vi "AUTO - TRANSLATE.vi"(8 "error in (no error)":errorcluster, 11 "auto pgm step":T2={"auto drive command"={"TRANSLATE"={"drive\ndistance (ft)"=0.0, "steer\nbearing (deg)"=0.0, "max strafe\nvelocity (ft/s)"=0.0, "max strafe\naccel (ft/s^2)"=58.7}, "ROTATE"={"rotate to\nbearing (deg)"=0.0, "max rotate\nvelocity (deg/s)"=0.0, "max rotate\naccel (ft/s^2)"=25.0}}, "sub-systems"={"start INTAKE"=FALSE, "extend FLAP"=FALSE, "SHOOT"=FALSE, "retract FLAP"=FALSE, "TARGET SPEAKER"=FALSE, "TARGET AMP"=FALSE, "TARGET OFF"=FALSE, "DANCE"=FALSE}} {"auto drive command"."ROTATE"."max rotate\naccel (ft/s^2)" min=0.0 max=200.0 step=0.1 format="%_3f"; "auto drive command"."ROTATE"."max rotate\nvelocity (deg/s)" min=0.0 step=0.001; "auto drive command"."TRANSLATE"."max strafe\naccel (ft/s^2)" min=0.0 max=200.0 step=0.1 format="%_3f"; "auto drive command"."TRANSLATE"."max strafe\nvelocity (ft/s)" min=0.0 max=20.0 step=0.001 format="%_5f"}) -> (0 "error out":errorcluster)   [LabVIEW 2023]
uses:
  ctrl defs/ctrl AUTONOMOUS step control.ctl
  ctrl defs/ctrl AUTONOMOUS drive step control.ctl
  ctrl defs/ctrl AUTONOMOUS systems step control.ctl
  <vilib>/Rock Robotics/WPI/ThirdParty/REV Robotics/REVLib/Typedef/Spark MAX Control Type.ctl
  Global INIT.vi
  Global odometry.vi
  <vilib>/addons/control/pid/pid.llb/PID (DBL).vi
  <vilib>/Rock Robotics/WPI/ThirdParty/Phoenix-LabVIEW/CANCoder/Get/CTRE_Phoenix_CANcoder_GetSensorData.vi
  <vilib>/addons/control/pid/NI_PID_pid.lvlib
panel:
  out "Yaw delta":dbl
  out "steer":dbl
  out "course\ncorrect\n(deg)":dbl
  in  "invert correction":bool
  out "err tol (in)":dbl
  in  "PID gains":T1={"proportional gain (Kc)"=1.0, "integral time (Ti, min)"=0.0, "derivative time (Td, min)"=0.0} {"derivative time (Td, min)" format="%.3f"; "integral time (Ti, min)" format="%.3f"; "proportional gain (Kc)" format="%.3f"}
  in  "output range":cluster{"output high":dbl, "output low":dbl}={"output high"=10.0, "output low"=-10.0} {"output low" format="%.2f"; "output high" format="%.2f"}
  out "auto drive command.TRANSLATE.steer\nbearing (deg)":dbl
  out "Yaw CURRENT":dbl
  out "Yaw init":dbl
  out "wheel\npos (rev)":dbl[](array[numeric])
  out "@ target":bool[](array[boolean])
  out "pos\ntarget (rev)":dbl[](array[numeric])
  out "rev tol\nto target":dbl
  out "distance (ft)\nto wheel revs":dbl
  out "vel to wheel\nspeed\n(rpm per ft/s)":dbl
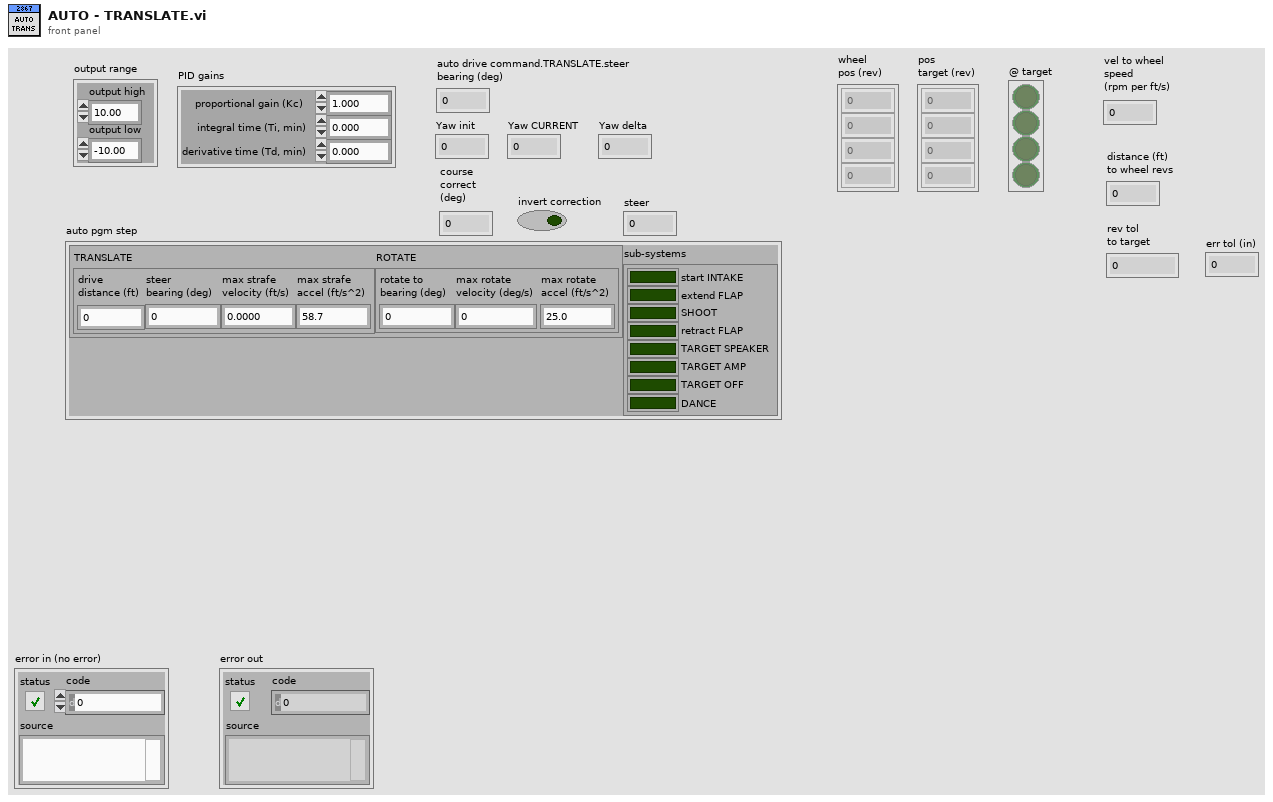
[diagram p1: front panel]
types:
  T1 = cluster{"proportional gain (Kc)":dbl, "integral time (Ti, min)":dbl, "derivative time (Td, min)":dbl}
  T2 = typedef "ctrl AUTONOMOUS step control.ctl" = cluster{"auto drive command":T3, "sub-systems":T4}
  T3 = typedef "ctrl AUTONOMOUS drive step control.ctl" = cluster{"TRANSLATE":cluster{"drive\ndistance (ft)":dbl, "steer\nbearing (deg)":dbl, "max strafe\nvelocity (ft/s)":dbl, "max strafe\naccel (ft/s^2)":dbl}, "ROTATE":cluster{"rotate to\nbearing (deg)":dbl, "max rotate\nvelocity (deg/s)":dbl, "max rotate\naccel (ft/s^2)":dbl}}
  T4 = typedef "ctrl AUTONOMOUS systems step control.ctl" = cluster{"start INTAKE":bool, "extend FLAP":bool, "SHOOT":bool, "retract FLAP":bool, "TARGET SPEAKER":bool, "TARGET AMP":bool, "TARGET OFF":bool, "DANCE":bool}
  T5 = typedef "WPI_MotorControlDeviceRef.ctl" = cluster{"DeviceStatus":errorcluster, "Type":T6, "PWM":cluster{"PWM Channel":T7, "DeadBand":T8}, "CAN":cluster{"Device Number":u8, "SetOutput VI Ref":variant, "GetOutput VI Ref":variant, "Enable VI Ref":variant, "Disable VI Ref":variant, "Data":variant}, "Invert":bool, "DIO PWM":cluster{"PWM \"Enable\" Channel":T7, "DIOChannel":T9, "PWM Rate":dbl}}
  T6 = typedef "WPI_MotorControlType.ctl" = enum16{"PWM", "CAN", "DIO PWM"}
  T7 = typedef "FPGA_DIOPWMChannel.ctl" = enum8{"PWM 0", "PWM 1", "PWM 2", "PWM 3", "PWM 4", "PWM 5", "PWM 6", "PWM 7", "PWM 8", "PWM 9", "PWM MXP 0", "PWM MXP 1", "PWM MXP 2", "PWM MXP 3", "PWM MXP 4", "PWM MXP 5", "PWM MXP 6", "PWM MXP 7", "PWM MXP 8", "PWM MXP 9", "Invalid"}
  T8 = typedef "WPI_PWMDeadband.ctl" = cluster{"Name":string, "maxPositivePwm":i32, "minPositivePwm":i32, "centerPwm":i32, "maxNegativePwm":i32, "minNegativePwm":i32, "angularRange":u16}
  T9 = typedef "FPGA_DIOChannel.ctl" = enum8{"DIO 0", "DIO 1", "DIO 2", "DIO 3", "DIO 4", "DIO 5", "DIO 6", "DIO 7", "DIO 8", "DIO 9", "DIO MXP 0", "DIO MXP 1", "DIO MXP 2", "DIO MXP 3", "DIO MXP 4", "DIO MXP 5", "DIO MXP 6", "DIO MXP 7", "DIO MXP 8", "DIO MXP 9", "DIO MXP 10", "DIO MXP 11", "DIO MXP 12", "DIO MXP 13", "DIO MXP 14", "DIO MXP 15", "SPI Port CS1", "SPI Port CS2", "SPI Port CS3", "SPI Port MISO", "SPI Port MOSI", "Invalid"}
  T10 = typedef "CTRE_Phoenix_CANcoder_DeviceRef.ctl" = cluster{"DeviceStatus":errorcluster, "Device Number":u8, "Handle":u64, "UsageFrame":u32, "Library Path":path}
  T11 = cluster{"Driver":T5, "Steer":T5, "Encoder":T10}[]
  T12 = cluster{"Rollover":dbl, "Yaw":dbl, "Cont Yaw":dbl}
  T13 = typedef "ctrl swerve motor.ctl" = cluster{"description":string, "MOTOR SELECT":T14, "Installed?":bool, "CAN ID":u8, "refnum name":string, "Invert":bool, "Idle Mode":T15, "Current limiting":T16, "MOTOR PIDF coefficients":T17, "gear ratio":dbl}
  T14 = typedef "ctrl MOTOR SELECT.ctl" = i16
  T15 = typedef "Spark MAX Idle Mode.ctl" = enum16{"Coast", "Brake"}
  T16 = typedef "ctrl Spark MAX current limiting.ctl" = cluster{"Linearized":bool, "Free Speed (A)":dbl, "Primay (A)":dbl, "Limit RPM (0)":u32}
  T17 = typedef "ctrl motor PIDF coefficients.ctl" = cluster{"PIDF":cluster{"P Gain":dbl, "I Gain":dbl, "D Gain":dbl, "F Gain":dbl, "I Zone":dbl, "Min Output":dbl, "Max Output":dbl}, "Smart Motion":T18}
  T18 = typedef "Spark MAX Smart Motion Parameters.ctl" = cluster{"Max Velocity":dbl, "Max Acceleration":dbl, "Minimum Velocity Output":dbl, "Allowed Closed Loop Error":dbl}
  T19 = typedef "ctrl swerve module.ctl" = cluster{"descr":string, "V":dbl, "POS":dbl, "target":dbl, "ABS":dbl, "from pivot to module":cluster{"R":dbl, "theta (deg)":dbl, "theta spin (deg)":dbl, "theta park (deg)":dbl}, "coord wrt geom CTR":cluster{"X":dbl, "Y":dbl}, "corner wt (lbm)":dbl}
  T20 = typedef "Spark MAX Control Type.ctl" = enum16{"Percent VBus", "Voltage", "Velocity", "Position", "Smart Motion", "Current", "Smart Velocity"}
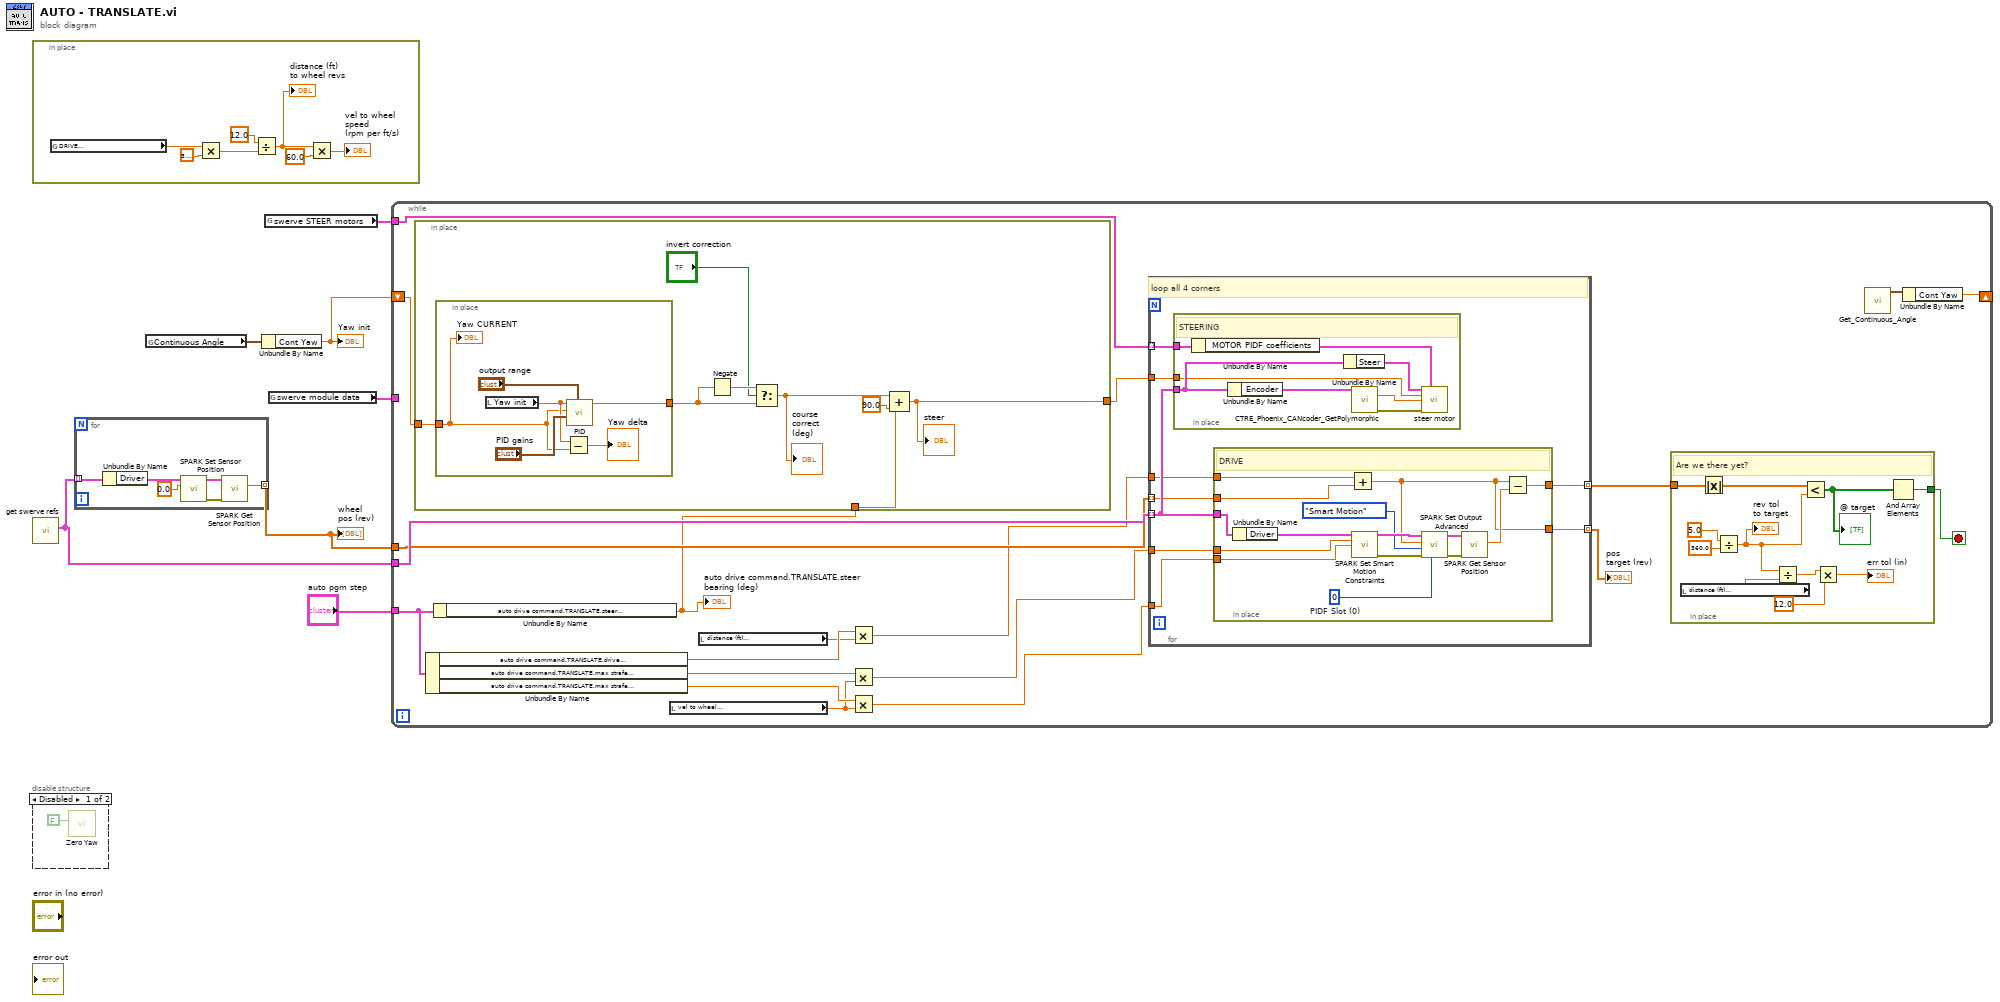
[diagram p0: block diagram]
diagram:
  n1 = in-place {
    n2 = global read "Global INIT.vi" "DRIVE\nwheel diam (in)"() -> (w14:dbl)
    n3 = Multiply(x=w14, y=3.141592653589793) -> (x*y=w11:dbl)
    n4 = Divide(x=12.0, y=w11) -> (x/y=w10:dbl)
    "distance (ft)\nto wheel revs" <- w10
    n5 = Multiply(x=w10, y=60.0) -> (x*y=→"vel to wheel\nspeed\n(rpm per ft/s)":dbl)
  }
  n6 = call "get swerve refs.vi"() -> ("Swerve refs"=w6:T11)  [unwired: 10 in, 1 out]
  n7 = disable-structure shown="Disabled" {
    frame Disabled {
      n8 = call <vilib>:"Zero Yaw.vi"("Zero"=FALSE) -> ()  [unwired: 11 in]
    }
    frame Enabled {
    }
  }
  n9 = for {
    tunnel: w6 -> [w21] mode=indexing
    tunnel: [w19] -> w3 mode=indexing
    n10 = Unbundle By Name(w21) -> ("Driver"=w20:T5)
    n11 = call <vilib>:"SPARK Set Sensor Position.vi"("Position"=0.0, "MotorControlDeviceRef"=w20) -> ("error out"=w17:errorcluster, "MotorControlDeviceRef"=w18:T5)  [unwired: 8 in]
    n12 = call <vilib>:"SPARK Get Sensor Position.vi"("error in (no error)"=w17, "MotorControlDevRef in"=w18) -> ("Sensor Position"=w19:dbl)  [unwired: 6 in, 3 out]
  }
  "wheel\npos (rev)" <- w3
  n13 = global read "Global odometry.vi" "Continuous Angle"() -> (w2:T12)
  n14 = Unbundle By Name(w2) -> ("Cont Yaw"=w1:dbl)
  "Yaw init" <- w1
  n15 = global read "Global INIT.vi" "swerve STEER motors"() -> (w5:T13[])
  n16 = global read "Global odometry.vi" "swerve module data"() -> (w4:T19[])
  n17 = while {
    tunnel: w3 -> [w39]
    tunnel: "auto pgm step" -> [w41]
    tunnel: w6 -> [w40]
    tunnel: w5 -> [w38]
    tunnel: w4 -> [_]
    shift-right: [w22] -> _
    shift-left: w1 -> [w25]
    stop <- w26 stop-if-true
    n18 = Unbundle By Name(w41) -> ("auto drive command.TRANSLATE.drive\ndistance (ft)"=w36:dbl, "auto drive command.TRANSLATE.max strafe\nvelocity (ft/s)"=w35:dbl, "auto drive command.TRANSLATE.max strafe\naccel (ft/s^2)"=w30:dbl)
    n19 = Unbundle By Name(w41) -> ("auto drive command.TRANSLATE.steer\nbearing (deg)"=w24:dbl)
    "auto drive command.TRANSLATE.steer\nbearing (deg)" <- w24
    n20 = in-place {
      in-place-border: [w49] -> w37
      in-place-border: w25 -> [w48]
      in-place-border: w24 -> [w47]
      n21 = in-place {
        in-place-border: w48 -> [w51]
        in-place-border: [w53] -> w44
        n22 = local read "Yaw init"() -> (w52:dbl)
        n23 = Subtract(x=w52, y=w51) -> (x-y=→"Yaw delta":dbl)
        n24 = call-poly <vilib>:"PID.vi"("output range"="output range", "PID gains"="PID gains", "process variable"=w51, "setpoint"=w52) -> ("output"=w53:dbl)  [unwired: 6 in, 1 out]
        "Yaw CURRENT" <- w51
      }
      n25 = Negate(x=w44) -> (-x=w43:dbl)
      n26 = Select(t=w43, s="invert correction", f=w44) -> (s? t:f=w45:dbl)
      "course\ncorrect\n(deg)" <- w45
      n27 = Compound Arithmetic op=ADD(w45, w47, 90.0 ("y")) -> (w49:dbl)
      "steer" <- w49
    }
    n28 = local read "vel to wheel\nspeed\n(rpm per ft/s)"() -> (w29:dbl)
    n29 = local read "distance (ft)\nto wheel revs"() -> (w34:dbl)
    n30 = Multiply(x=w36, y=w34) -> (x*y=w33:dbl)
    n31 = Multiply(x=w35, y=w29) -> (x*y=w32:dbl)
    n32 = Multiply(x=w30, y=w29) -> (x*y=w31:dbl)
    n33 = for {
      tunnel: w40 -> [w73] mode=indexing
      tunnel: w39 -> [w69] mode=indexing
      tunnel: w38 -> [w74] mode=indexing
      tunnel: w37 -> [w75]
      tunnel: w33 -> [w72]
      tunnel: w32 -> [w70]
      tunnel: w31 -> [w71]
      tunnel: [w68] -> w28 mode=indexing
      tunnel: [w67] -> w27 mode=indexing
      # "loop all 4 corners"
      n34 = in-place {
        in-place-border: w73 -> [w95]
        in-place-border: w75 -> [w94]
        in-place-border: w74 -> [w92]
        # "STEERING"
        n35 = Unbundle By Name(w92) -> ("MOTOR PIDF coefficients"=w91:T17)
        n36 = Unbundle By Name(w95) -> ("Encoder"=w98:T10)
        n37 = Unbundle By Name(w95) -> ("Steer"=w96:T5)
        n38 = call-poly <vilib>:"CTRE_Phoenix_CANcoder_GetPolymorphic.vi"("CTRE_CANcoder_DeviceRef"=w98) -> ("Position"=w97:dbl, "error out"=w93:errorcluster)  [unwired: 10 in, 3 out]
        n39 = call "steer motor.vi"("MotorControlDevRef"=w96, "MOTOR PIDF coefficients"=w91, "target"=w94, "encoder"=w97, "error in (no error)"=w93) -> ()  [unwired: 10 in, 1 out]
      }
      n40 = in-place {
        in-place-border: w73 -> [w86]
        in-place-border: w72 -> [w84]
        in-place-border: w71 -> [w82]
        in-place-border: w70 -> [w83]
        in-place-border: w69 -> [w81]
        in-place-border: [w77] -> w68
        in-place-border: [w76] -> w67
        w87 = 0  # PIDF Slot (0)
        # "DRIVE"
        n41 = Unbundle By Name(w86) -> ("Driver"=w85:T5)
        n42 = Add(x=w84, y=w81) -> (x+y=w76:dbl)
        n43 = call <vilib>:"SPARK Set Smart Motion Constraints.vi"("MotorControlDeviceRef"=w85, "Max Velocity"=w83, "Max Acceleration"=w82) -> ("MotorControlDeviceRef"=w89:T5, "error out"=w90:errorcluster)  [unwired: 11 in]
        n44 = call <vilib>:"SPARK Set Output Advanced.vi"("PIDF Slot (0)"=w87, "error in (no error)"=w90, "Control Mode"=Spark_MAX_Control_Type."Smart Motion", "Setpoint"=w76, "MotorControlDevRef"=w89) -> ("error out"=w80:errorcluster, "MotorControlDevRef"=w79:T5)  [unwired: 5 in]
        n45 = call <vilib>:"SPARK Get Sensor Position.vi"("error in (no error)"=w80, "MotorControlDevRef in"=w79) -> ("Sensor Position"=w78:dbl)  [unwired: 6 in, 3 out]
        n46 = Subtract(x=w76, y=w78) -> (x-y=w77:dbl)
      }
    }
    "pos\ntarget (rev)" <- w27
    n47 = in-place {
      in-place-border: w28 -> [w66]
      in-place-border: [w61] -> w26
      # "Are we there yet?"
      n48 = local read "distance (ft)\nto wheel revs"() -> (w59:dbl)
      n49 = Absolute Value(x=w66) -> (abs(x)=w65:dbl[])
      n50 = Divide(x=5.0, y=360.0) -> (x/y=w60:dbl)
      "rev tol\nto target" <- w60
      n51 = Divide(x=w60, y=w59) -> (x/y=w58:dbl)
      n52 = Less?(x=w65, y=w60) -> (x < y?=w62:bool[])
      "@ target" <- w62
      n53 = Multiply(x=w58, y=12.0) -> (x*y=→"err tol (in)":dbl)
      n54 = And Array Elements(Boolean array=w62) -> (logical AND=w61:bool)
    }
    n55 = call <vilib>:"Get_Continuous_Angle.vi"() -> ("Continuous Angle"=w23:T12)  [unwired: 11 in]
    n56 = Unbundle By Name(w23) -> ("Cont Yaw"=w22:dbl)
  }
